vi "Autonomous Independent.vi"() -> ()   [LabVIEW 2017]
doc: "This VI is called when autonomous begins, and will automatically be terminated when autonomous ends. You can carry out timed or sensor driven robot movement independently without needing to return to the caller."
uses:
  <vilib>/Rock Robotics/WPI/ThirdParty/Sensors/navX/_TypeDefs/FRIC_navX_DeviceNumbersTypeDef.ctl
  <vilib>/Rock Robotics/WPI/Solenoid/WPI_SolenoidValue.ctl
  <vilib>/Rock Robotics/WPI/ThirdParty/Phoenix-LabVIEW/Motor Controller/Controls/CTRE_Phoenix_MotorControl_ControlMode.ctl
  <vilib>/Rock Robotics/WPI/Utilities/WPI_GetSetVariantRefNum.vi
  <vilib>/Rock Robotics/Network Tables/NT Read String.vi
  <vilib>/Rock Robotics/Network Tables/NT Write Numeric Array.vi
  <vilib>/Rock Robotics/WPI/Solenoid/WPI_SolenoidSetEnum.vi
panel:
  out "error out":errorcluster
  out "Array":dbl[](array[numeric])
  out "Direction":string[](array[string])
  in  "Target Angle":dbl format="%#_13g"
  in  "Target Distance":dbl=500.0 format="%#_13g"
  # "Be sure to right-click and choose Data Operations>>Make Current Value default if you want to save the array values with the VI"
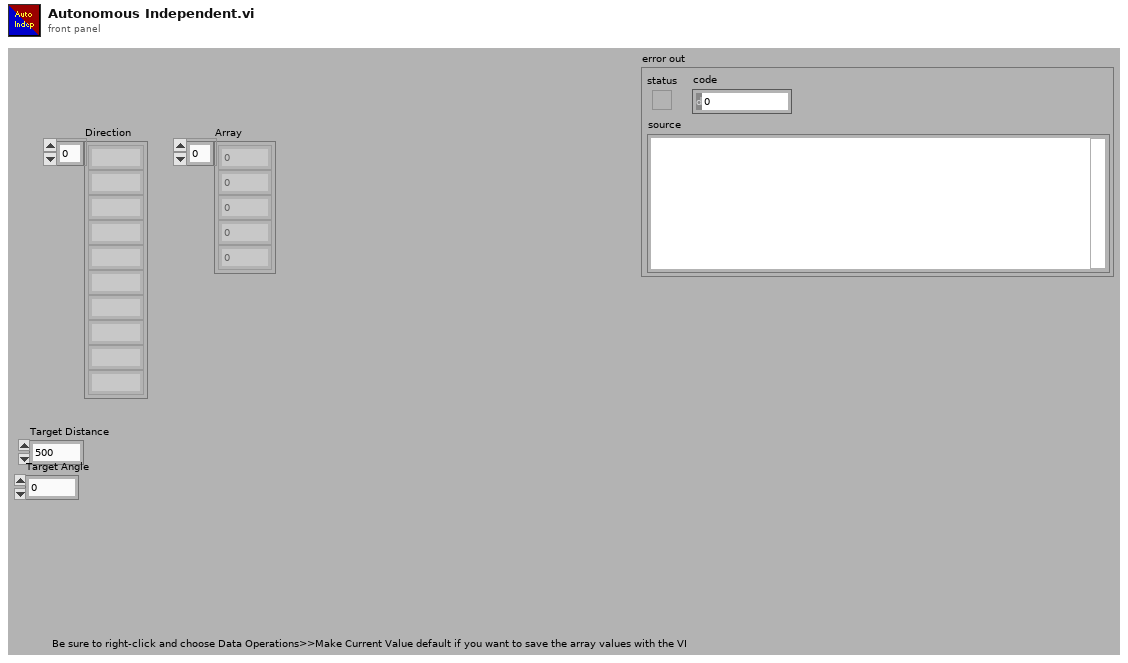
[diagram p1: front panel]
types:
  T1 = typedef "FRIC_navX_DeviceNumbersTypeDef.ctl" = enum16{"Dev0", "Dev1", "Dev2", "Dev3"}
  T2 = cluster{"Left Encoder":string, "Right Encoder":string, "Gyro Refnum":string, "Device Number":T1, "Right Refnum":string, "Left Refnum":string, "Right Intake":string, "Left Intake":string}
  T3 = typedef "WPI_JoystickDevRef.ctl" = cluster{"Device":T4}
  T4 = typedef "WPI_JoystickDeviceEnum.ctl" = enum16{"USB 0", "USB 1", "USB 2", "USB 3", "USB 4", "USB 5"}
  T5 = typedef "WPI_SolenoidValue.ctl" = enum16{"Off", "On", "Forward", "Reverse"}
  T6 = typedef "WPI_SolenoidDevRef.ctl" = cluster{"DevStatus":errorcluster, "Pneumatics Control Module":u8, "Forward Solenoid Channel":T7, "Reverse Solenoid Channel":T7}
  T7 = typedef "WPI_SolenoidChannel.ctl" = enum8{"Solenoid 0", "Solenoid 1", "Solenoid 2", "Solenoid 3", "Solenoid 4", "Solenoid 5", "Solenoid 6", "Solenoid 7", "Invalid"}
  T8 = cluster{"Left Encoder":string, "Right Encoder":string, "Gyro Refnum":string, "Device Number":T1, "Right Refnum":string, "Left Refnum":string}
  T9 = cluster{"Left Encoder":string, "Right Encoder":string, "Gyro Refnum":string, "Device Number":T1, "Right Refnum":string, "Left Refnum":string, "Left Intake":string, "Right Intake":string}
  T10 = typedef "CTRE_Phoenix_MotorControl_ControlMode.ctl" = u16
  T11 = typedef "WPI_MotorControlDeviceRef.ctl" = cluster{"DeviceStatus":errorcluster, "Type":T12, "PWM":cluster{"PWM Channel":T13, "DeadBand":T14}, "CAN":cluster{"Device Number":u8, "SetOutput VI Ref":variant, "GetOutput VI Ref":variant, "Enable VI Ref":variant, "Disable VI Ref":variant, "Data":variant}, "Invert":bool, "DIO PWM":cluster{"PWM \"Enable\" Channel":T13, "DIOChannel":T15, "PWM Rate":dbl}}
  T12 = typedef "WPI_MotorControlType.ctl" = enum16{"PWM", "CAN", "DIO PWM"}
  T13 = typedef "FPGA_DIOPWMChannel.ctl" = enum8{"PWM 0", "PWM 1", "PWM 2", "PWM 3", "PWM 4", "PWM 5", "PWM 6", "PWM 7", "PWM 8", "PWM 9", "PWM MXP 0", "PWM MXP 1", "PWM MXP 2", "PWM MXP 3", "PWM MXP 4", "PWM MXP 5", "PWM MXP 6", "PWM MXP 7", "PWM MXP 8", "PWM MXP 9", "Invalid"}
  T14 = typedef "WPI_PWMDeadband.ctl" = cluster{"Name":string, "maxPositivePwm":i32, "minPositivePwm":i32, "centerPwm":i32, "maxNegativePwm":i32, "minNegativePwm":i32, "angularRange":u16}
  T15 = typedef "FPGA_DIOChannel.ctl" = enum8{"DIO 0", "DIO 1", "DIO 2", "DIO 3", "DIO 4", "DIO 5", "DIO 6", "DIO 7", "DIO 8", "DIO 9", "DIO MXP 0", "DIO MXP 1", "DIO MXP 2", "DIO MXP 3", "DIO MXP 4", "DIO MXP 5", "DIO MXP 6", "DIO MXP 7", "DIO MXP 8", "DIO MXP 9", "DIO MXP 10", "DIO MXP 11", "DIO MXP 12", "DIO MXP 13", "DIO MXP 14", "DIO MXP 15", "SPI Port CS1", "SPI Port CS2", "SPI Port CS3", "SPI Port MISO", "SPI Port MOSI", "Invalid"}
  T16 = cluster{"Width":u16, "Style":enum32{"Solid", "Dash", "Dot", "DashDot", "DashDotDot"}}
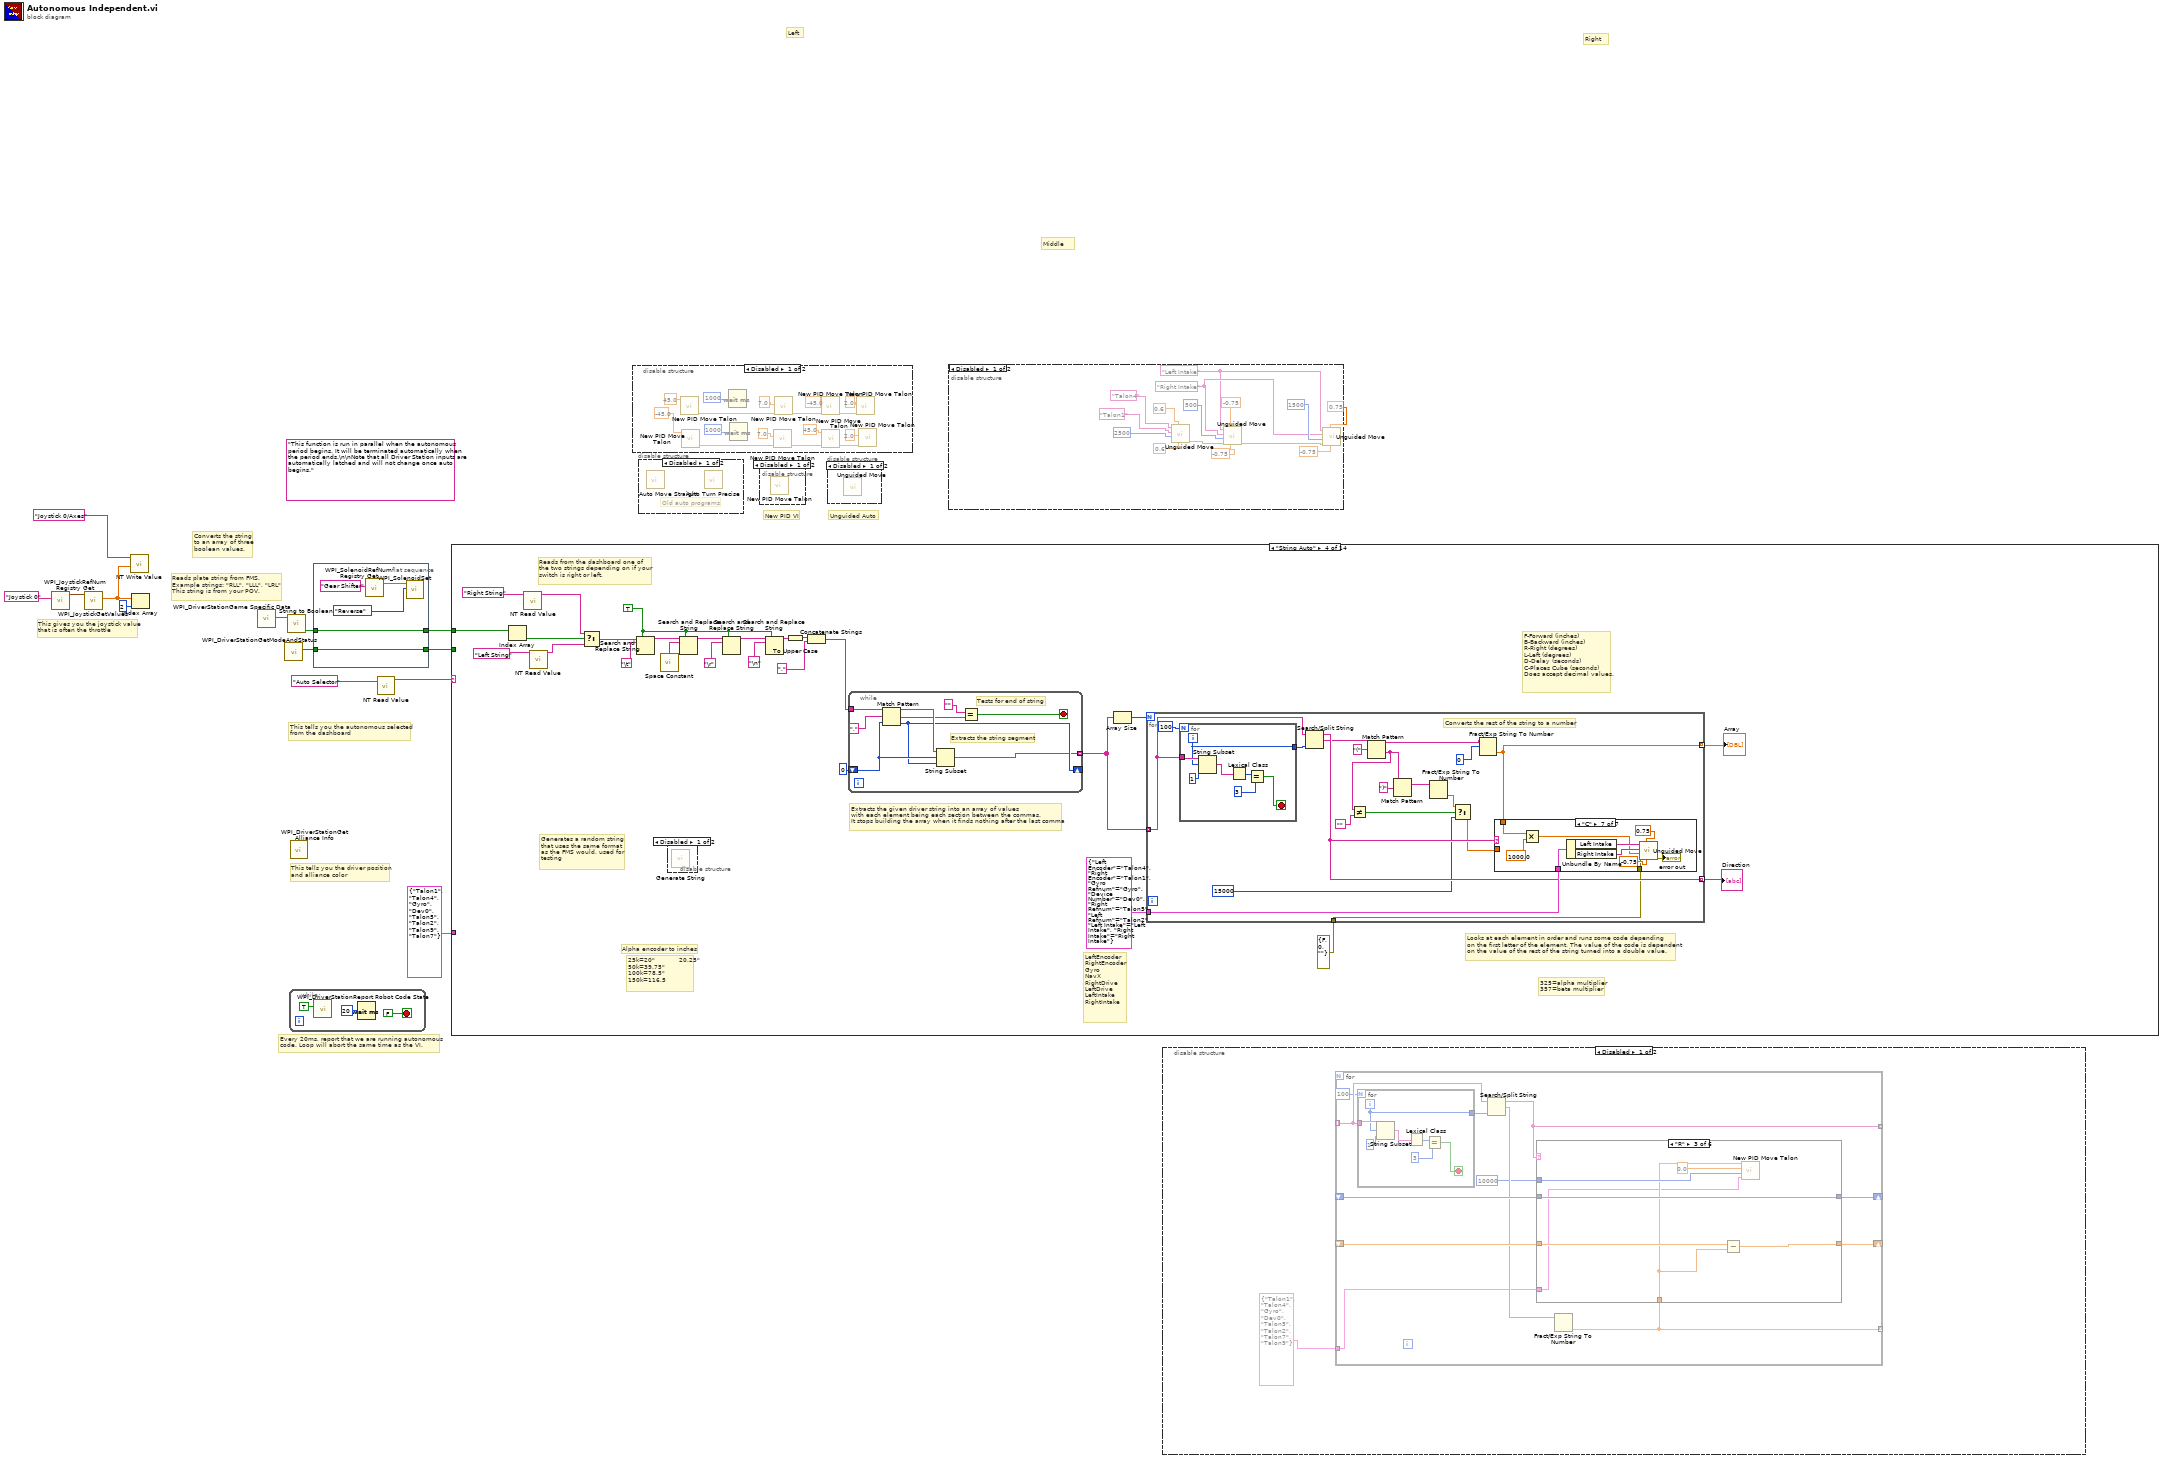
[diagram p0: block diagram]
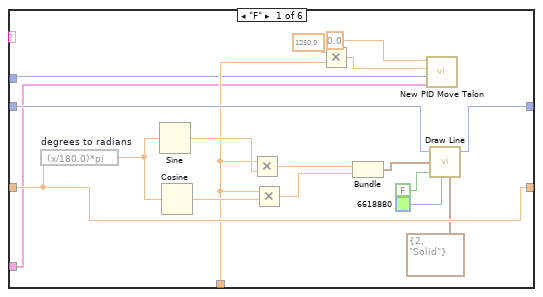
[diagram p2: hidden frame]
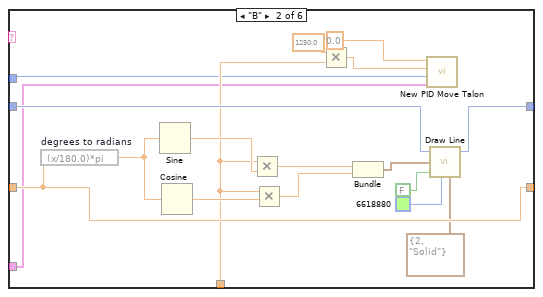
[diagram p3: hidden frame]
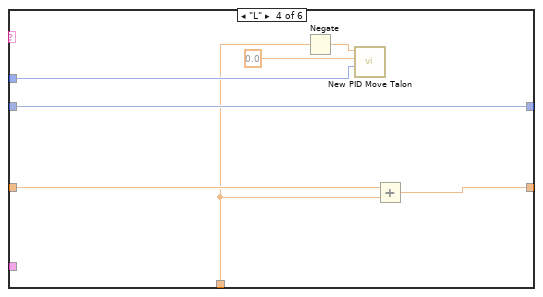
[diagram p4: hidden frame]
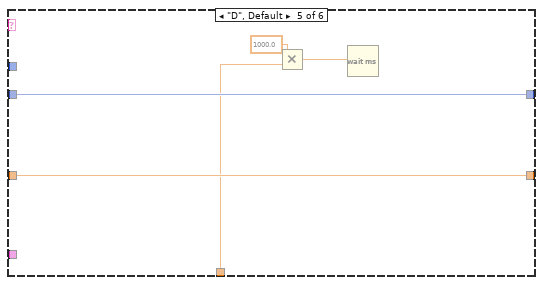
[diagram p5: hidden frame]
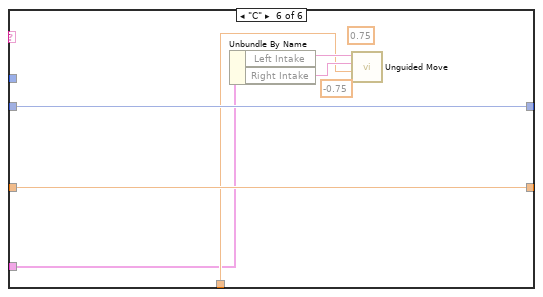
[diagram p6: hidden frame]
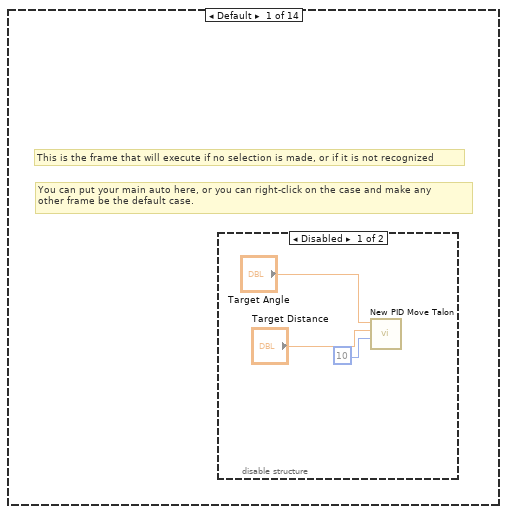
[diagram p13: hidden frame]
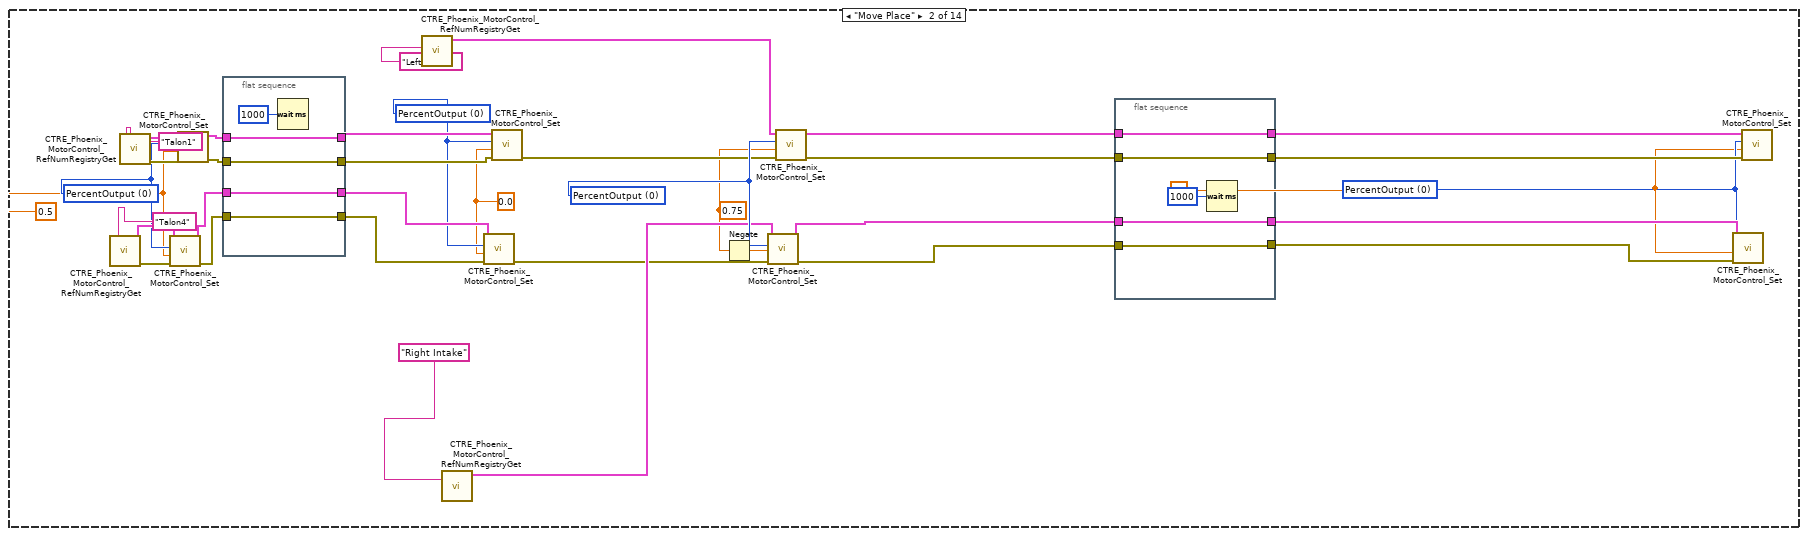
[diagram p15: hidden frame]
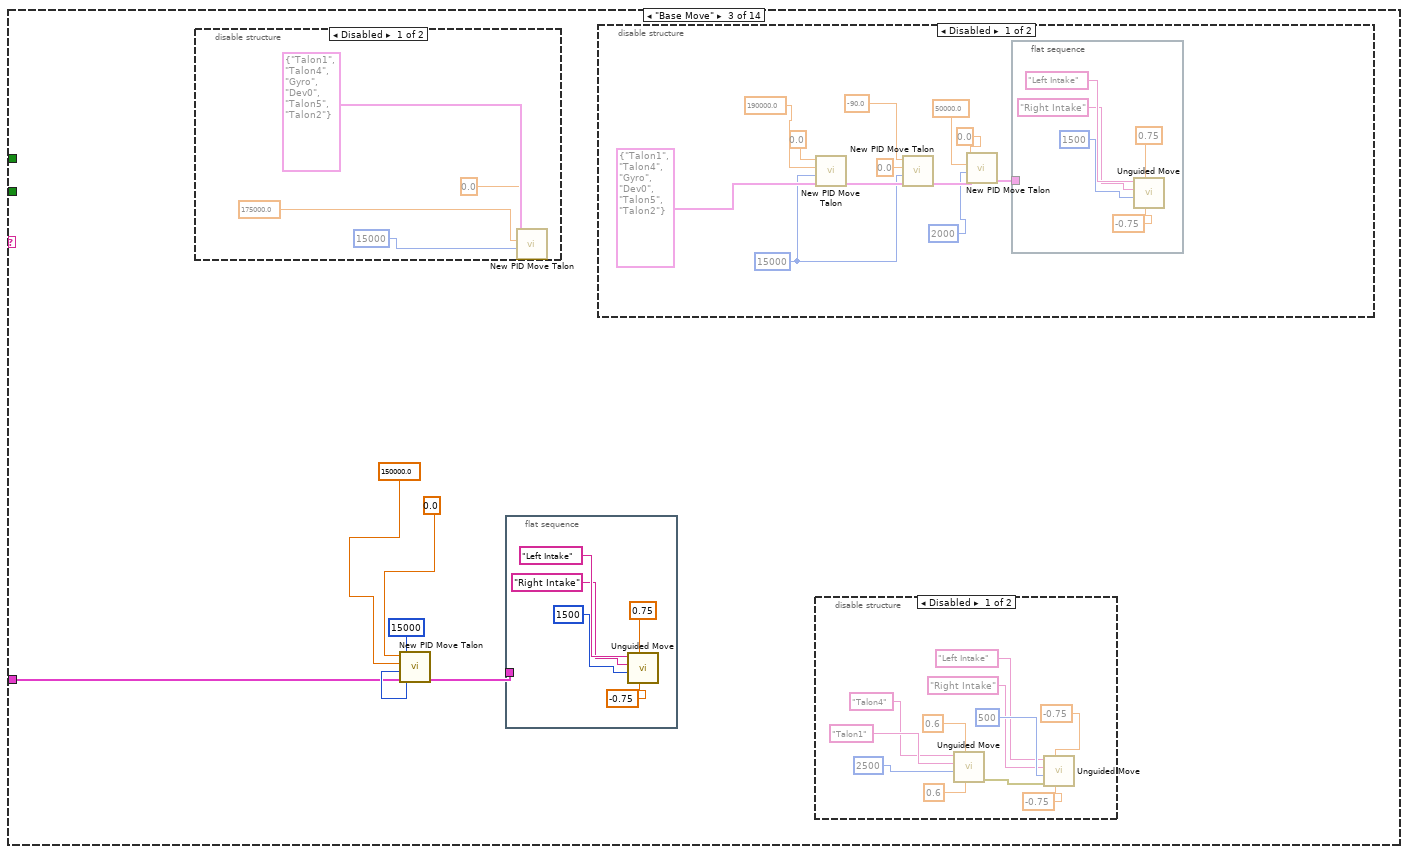
[diagram p16: hidden frame]
diagram:
  (unwired) "This function is run in parallel when the autonomous period begins. It will be terminated automatically when the period ends.\n\nNote that all Driver Station inputs are automatically latched and will not change once auto begins."
  # "Unguided Auto"
  # "New PID VI"
  # "Converts the string\nto an array of three\nboolean values."
  # "Reads plate string from FMS. \nExample strings: \"RLL\", \"LLL\", \"LRL\"\nThis string is from your POV."
  # "Middle"
  # "Left"
  # "Right"
  # "This tells you the autonomous selected\nfrom the dashboard"
  # "Every 20ms, report that we are running autonomous\ncode. Loop will abort the same time as the VI."
  # "This gives you the joystick value\nthat is often the throttle"
  # "This tells you the driver position\nand alliance color"
  n1 = call <vilib>:"WPI_JoystickRefNum Registry Get.vi"("refnum name"="Joystick 0") -> ("JoystickDevRef"=w12:T3)  [unwired: 1 in, 9 out]
  n2 = call <vilib>:"WPI_JoystickGetValues.vi"("JoystickDevRef"=w12) -> ("Axes"=w8:dbl[])  [unwired: 6 in, 4 out]
  n3 = call-poly <vilib>:"NT Write Value.vi"("Numeric Array"=w8, "Name"="Joystick 0/Axes") -> ()  [unwired: 9 in, 1 out]
  n4 = Index Array(array=w8, index=2) -> ()  [unwired: 1 out]
  n5 = call <vilib>:"WPI_DriverStationGame Specific Data.vi"() -> ("Game Specific Data"=w6:string)  [unwired: 11 in]
  n6 = call <vilib>:"WPI_DriverStationGetModeAndStatus.vi"() -> ("FMS Attached"=w1:bool)  [unwired: 10 in, 1 out]
  n7 = call "String to Boolean.vi"("String"=w6) -> ("Boolean Array"=w3:bool[])  [unwired: 10 in]
  n8 = while {
    stop <- FALSE stop-if-true
    n9 = call <vilib>:"WPI_DriverStationReport Robot Code State.vi"("Autonomous"=TRUE) -> ()  [unwired: 10 in, 1 out]
    n10 = Wait (ms)(milliseconds to wait=u32 20) -> ()  [unwired: 1 out]
  }
  n11 = call <vilib>:"WPI_DriverStationGet Alliance Info.vi"() -> ()  [unwired: 12 out]
  n12 = flat-sequence {
    tunnel: [w21] -> w4
    tunnel: w3 -> [w21]
    tunnel: [w17] -> w2
    tunnel: w1 -> [w17]
    frame #0 {
      n13 = call <vilib>:"WPI_SolenoidRefNum Registry Get.vi"("refnum name"="Gear Shifter") -> ("SolenoidDevRef"=w20:T6)  [unwired: 9 in, 1 out]
      n14 = call-poly <vilib>:"WPI_SolenoidSet.vi"("Value"=WPI_SolenoidValue."Reverse", "SolenoidDevRef"=w20) -> ()  [unwired: 8 in, 2 out]
    }
  }
  n15 = call-poly <vilib>:"NT Read Value.vi"("Name"="Auto Selector") -> ("String"=w9:string)  [unwired: 9 in, 1 out]
  n16 = case shown="\"String Auto\"" w9 {
    tunnel: w4 -> [_ _ _ w128 w212 _ _ w260 _ _ _ _ _ _]
    tunnel: T2 {"Left Encoder"="Talon1", "Right Encoder"="Talon4", "Gyro Refnum"="Gyro", "Device Number"=enum."Dev0", "Right Refnum"="Talon5", "Left Refnum"="Talon2", "Right Intake"="Talon9", "Left Intake"="Talon7"} ("Cluster 3") -> [_ _ w72 _ _ _ _ _ _ _ _ _ _ _]
    tunnel: w2 -> [_ _ _ _ _ _ _ _ _ _ _ _ _ _]
    frame Default {
      # "You can put your main auto here, or you can right-click on the case and make any\nother frame be the default case."
      # "This is the frame that will execute if no selection is made, or if it is not recognized"
      n17 = disable-structure shown="Disabled" {
        frame Disabled {
          n18 = call "New PID Move Talon.vi"("Timeout"=i8 10, "Target Distance"="Target Distance", "Target Angle"="Target Angle") -> ()  [unwired: 8 in, 1 out]
        }
        frame Enabled {
        }
      }
    }
    frame "Move Place" {
      w27 = 0.0 ("Output")
      w28 = T10 0 items=["PercentOutput"=0, "Position"=1, "Velocity"=2, "Current"=3, "Follower"=5, "MotionProfile"=6, "MotionMagic"=7, "MotionMagicArc"=8, "MotionProfileArc"=10, "Disabled"=15] ("Control Mode")
      w26 = 0.75 ("Output")
      w43 = T10 0 items=["PercentOutput"=0, "Position"=1, "Velocity"=2, "Current"=3, "Follower"=5, "MotionProfile"=6, "MotionMagic"=7, "MotionMagicArc"=8, "MotionProfileArc"=10, "Disabled"=15] ("Control Mode")
      w44 = 0.0 ("Output")
      w45 = T10 0 items=["PercentOutput"=0, "Position"=1, "Velocity"=2, "Current"=3, "Follower"=5, "MotionProfile"=6, "MotionMagic"=7, "MotionMagicArc"=8, "MotionProfileArc"=10, "Disabled"=15] ("Control Mode")
      w54 = 0.5 ("Output")
      w55 = T10 0 items=["PercentOutput"=0, "Position"=1, "Velocity"=2, "Current"=3, "Follower"=5, "MotionProfile"=6, "MotionMagic"=7, "MotionMagicArc"=8, "MotionProfileArc"=10, "Disabled"=15] ("Control Mode")
      n19 = call <vilib>:"CTRE_Phoenix_MotorControl_RefNumRegistryGet.vi"("refnum name"="Talon4") -> ("error out"=w56:errorcluster, "PhoenixMotorControlDevRef"=w57:T11)  [unwired: 9 in]
      n20 = call <vilib>:"CTRE_Phoenix_MotorControl_RefNumRegistryGet.vi"("refnum name"="Talon1") -> ("error out"=w59:errorcluster, "PhoenixMotorControlDevRef"=w58:T11)  [unwired: 9 in]
      n21 = call <vilib>:"CTRE_Phoenix_MotorControl_Set.vi"("error in (no error)"=w56, "Output"=w54, "Control Mode"=w55, "PhoenixMotorControlDevRef"=w57) -> ("error out"=w50:errorcluster, "PhoenixMotorControlDevRef"=w51:T11)  [unwired: 6 in]
      n22 = call <vilib>:"CTRE_Phoenix_MotorControl_Set.vi"("error in (no error)"=w59, "Output"=w54, "Control Mode"=w55, "PhoenixMotorControlDevRef"=w58) -> ("error out"=w52:errorcluster, "PhoenixMotorControlDevRef"=w53:T11)  [unwired: 6 in]
      n23 = flat-sequence {
        tunnel: w53 -> [w71]
        tunnel: [w71] -> w49
        tunnel: [w70] -> w47
        tunnel: w51 -> [w70]
        tunnel: [w69] -> w46
        tunnel: w50 -> [w69]
        tunnel: w52 -> [w68]
        tunnel: [w68] -> w48
        frame #0 {
          n24 = Wait (ms)(milliseconds to wait=u32 1000) -> ()  [unwired: 1 out]
        }
      }
      n25 = call <vilib>:"CTRE_Phoenix_MotorControl_RefNumRegistryGet.vi"("refnum name"="Left Intake") -> ("PhoenixMotorControlDevRef"=w42:T11)  [unwired: 9 in, 1 out]
      n26 = call <vilib>:"CTRE_Phoenix_MotorControl_RefNumRegistryGet.vi"("refnum name"="Right Intake") -> ("PhoenixMotorControlDevRef"=w41:T11)  [unwired: 9 in, 1 out]
      n27 = call <vilib>:"CTRE_Phoenix_MotorControl_Set.vi"("error in (no error)"=w46, "Output"=w44, "Control Mode"=w45, "PhoenixMotorControlDevRef"=w47) -> ("error out"=w40:errorcluster)  [unwired: 6 in, 1 out]
      n28 = call <vilib>:"CTRE_Phoenix_MotorControl_Set.vi"("error in (no error)"=w48, "Output"=w44, "Control Mode"=w45, "PhoenixMotorControlDevRef"=w49) -> ("error out"=w39:errorcluster)  [unwired: 6 in, 1 out]
      n29 = Negate(x=w26) -> (-x=w25:dbl)
      n30 = call <vilib>:"CTRE_Phoenix_MotorControl_Set.vi"("error in (no error)"=w40, "Output"=w25, "Control Mode"=w43, "PhoenixMotorControlDevRef"=w41) -> ("error out"=w36:errorcluster, "PhoenixMotorControlDevRef"=w33:T11)  [unwired: 6 in]
      n31 = call <vilib>:"CTRE_Phoenix_MotorControl_Set.vi"("error in (no error)"=w39, "Output"=w26, "Control Mode"=w43, "PhoenixMotorControlDevRef"=w42) -> ("error out"=w35:errorcluster, "PhoenixMotorControlDevRef"=w34:T11)  [unwired: 6 in]
      n32 = flat-sequence {
        tunnel: [w66] -> w29
        tunnel: w36 -> [w66]
        tunnel: [w65] -> w31
        tunnel: w35 -> [w65]
        tunnel: [w64] -> w32
        tunnel: w34 -> [w64]
        tunnel: [w63] -> w30
        tunnel: w33 -> [w63]
        frame #0 {
          n33 = Wait (ms)(milliseconds to wait=u32 1000) -> ()  [unwired: 1 out]
        }
      }
      n34 = call <vilib>:"CTRE_Phoenix_MotorControl_Set.vi"("error in (no error)"=w29, "Output"=w27, "Control Mode"=w28, "PhoenixMotorControlDevRef"=w30) -> ()  [unwired: 6 in, 2 out]
      n35 = call <vilib>:"CTRE_Phoenix_MotorControl_Set.vi"("error in (no error)"=w31, "Output"=w27, "Control Mode"=w28, "PhoenixMotorControlDevRef"=w32) -> ()  [unwired: 6 in, 2 out]
    }
    frame "Base Move" {
      n36 = disable-structure shown="Disabled" {
        frame Disabled {
          n37 = call "New PID Move Talon.vi"("Cluster 3"=T8 {"Left Encoder"="Talon1", "Right Encoder"="Talon4", "Gyro Refnum"="Gyro", "Device Number"=enum."Dev0", "Right Refnum"="Talon5", "Left Refnum"="Talon2"}, "Timeout"=i16 15000, "Target Distance"=175000.0 ("Target Distance 2"), "Target Angle"=0.0) -> ()  [unwired: 7 in, 1 out]
        }
        frame Enabled {
        }
      }
      n38 = call "New PID Move Talon.vi"("Cluster 3"=w72, "Timeout"=i16 15000, "Target Distance"=150000.0, "Target Angle"=0.0) -> ("Cluster 2"=w73:T2)  [unwired: 7 in]
      n39 = flat-sequence {
        tunnel: w73 -> [_]
        frame #0 {
          n40 = call "Unguided Move.vi"("Power 2"=-0.75 ("Power"), "Power"=0.75, "milliseconds to wait"=u32 1500, "refnum name 2"="Right Intake" ("refnum name"), "refnum name"="Left Intake") -> ()  [unwired: 6 in, 1 out]
        }
      }
      n41 = disable-structure shown="Disabled" {
        frame Disabled {
          w89 = i16 15000 ("Timeout")
          n42 = call "New PID Move Talon.vi"("Cluster 3"=T8 {"Left Encoder"="Talon1", "Right Encoder"="Talon4", "Gyro Refnum"="Gyro", "Device Number"=enum."Dev0", "Right Refnum"="Talon5", "Left Refnum"="Talon2"}, "Timeout"=w89, "Target Distance"=190000.0, "Target Angle"=0.0) -> ("Cluster 2"=w93:T2)  [unwired: 7 in]
          n43 = call "New PID Move Talon.vi"("Cluster 3"=w93, "Timeout"=w89, "Target Distance"=0.0, "Target Angle"=-90.0) -> ("Cluster 2"=w92:T2)  [unwired: 7 in]
          n44 = call "New PID Move Talon.vi"("Cluster 3"=w92, "Timeout"=i16 2000, "Target Distance"=50000.0, "Target Angle"=0.0) -> ("Cluster 2"=w91:T2)  [unwired: 7 in]
          n45 = flat-sequence {
            tunnel: w91 -> [_]
            frame #0 {
              n46 = call "Unguided Move.vi"("Power 2"=-0.75 ("Power"), "Power"=0.75, "milliseconds to wait"=u32 1500, "refnum name 2"="Right Intake" ("refnum name"), "refnum name"="Left Intake") -> ()  [unwired: 6 in, 1 out]
            }
          }
        }
        frame Enabled {
        }
      }
      n47 = disable-structure shown="Disabled" {
        frame Disabled {
          n48 = call "Unguided Move.vi"("Power 2"=0.6, "Power"=0.6, "milliseconds to wait"=u32 2500, "refnum name 2"="Talon1", "refnum name"="Talon4") -> ("error out"=w109:errorcluster)  [unwired: 6 in]
          n49 = call "Unguided Move.vi"("Power 2"=-0.75 ("Power"), "Power"=-0.75, "error in (no error)"=w109, "milliseconds to wait"=u32 500, "refnum name 2"="Right Intake" ("refnum name"), "refnum name"="Left Intake") -> ()  [unwired: 5 in, 1 out]
        }
        frame Enabled {
        }
      }
    }
    frame "String Auto" {
      w120 = TRUE ("replace all? (F)")
      # "325=alpha multiplier\n357=beta multiplier"
      # "F-Forward (inches)\nB-Backward (inches)\nR-Right (degrees)\nL-Left (degrees)\nD-Delay (seconds)\nC-Places Cube (seconds)\nDoes accept decimal values."
      # "Alpha encoder to inches"
      # "LeftEncoder\nRightEncoder\nGyro\nNavX\nRightDrive\nLeftDrive\nLeftIntake\nRightIntake"
      # "25k=20\"            20.25\"\n50k=39.75\"\n100k=78.5\"\n150k=116.5"
      # "Looks at each element in order and runs some code depending\non the first letter of the element. The value of the code is dependent\non the value of the rest of the string turned into a double value."
      # "Extracts the given driver string into an array of values \nwith each element being each section between the commas.\nIt stops building the array when it finds nothing after the last comma"
      # "Reads from the dashboard one of\nthe two strings depending on if your\nswitch is right or left."
      # "Generates a random string\nthat uses the same format \nas the FMS would, used for\ntesting"
      n50 = Index Array(array=w128) -> (element=w139:bool)  [unwired: 1 in]
      n51 = call-poly <vilib>:"NT Read Value.vi"("Name"="Right String") -> ("String"=w138:string)  [unwired: 9 in, 1 out]
      n52 = call-poly <vilib>:"NT Read Value.vi"("Name"="Left String") -> ("String"=w135:string)  [unwired: 9 in, 1 out]
      n53 = Select(t=w138, s=w139, f=w135) -> (s? t:f=w118:string)
      n54 = Search and Replace String(replace all?=w120, input string=w118, search string="\t") -> (result string=w124:string)  [unwired: 5 in, 3 out]
      n55 = call <vilib>:"Space Constant.vi"() -> ("String"=w122:string)
      n56 = disable-structure shown="Disabled" {
        frame Disabled {
          n57 = call "Generate String.vi"() -> ()  [unwired: 11 in, 1 out]
        }
        frame Enabled {
        }
      }
      n58 = Search and Replace String(replace all?=w120, input string=w124, search string=w122) -> (result string=w125:string)  [unwired: 5 in, 3 out]
      n59 = Search and Replace String(replace all?=w120, input string=w125, search string="\r") -> (result string=w126:string)  [unwired: 5 in, 3 out]
      n60 = Search and Replace String(replace all?=w120, input string=w126, search string="\n") -> (result string=w119:string)  [unwired: 5 in, 3 out]
      n61 = To Upper Case(1:w119) -> (0:w116:string)
      n62 = Concatenate Strings(w116, "," ("regular expression")) -> (w115:string)
      n63 = while {
        tunnel: w115 -> [w209]
        shift-right: [w205] -> _
        shift-left: 0 ("offset past match") -> [w206]
        tunnel: [w204] -> w132 mode=indexing
        stop <- w201 stop-if-true
        # "Tests for end of string"
        # "Extracts the string segment"
        n64 = Match Pattern(string=w209, regular expression=",", offset (0)=w206) -> (before substring=w207:string, after substring=w203:string, offset past match=w205:i32)  [unwired: 1 out]
        n65 = String Subset(string=w207, offset (0)=w206, length (rest)=w205) -> (substring=w204:string)
        n66 = Equal?(x="", y=w203) -> (x = y?=w201:bool)
      }
      n67 = Array Size(array=w132) -> (size(s)=w133:i32)
      n68 = for {
        N: w133 -> [_]
        tunnel: w132 -> [w154] mode=indexing
        tunnel: [w157] -> w130 mode=indexing
        tunnel: [w153] -> w131 mode=indexing
        tunnel: T9 {"Left Encoder"="Talon4", "Right Encoder"="Talon1", "Gyro Refnum"="Gyro", "Device Number"=enum."Dev0", "Right Refnum"="Talon5", "Left Refnum"="Talon2", "Left Intake"="Left Intake", "Right Intake"="Right Intake"} ("Cluster 3") -> [w156]
        tunnel: errorcluster {"status"=FALSE, "code"=0, "source"=""} ("error in (no error)") -> [w151]
        # "Converts the rest of the string to a number"
        n69 = for {
          N: 100 -> [_]
          tunnel: w154 -> [w163]
          tunnel: [w160] -> w155
          i -> [w160]
          stop <- w159 stop-if-true
          n70 = String Subset(string=w163, offset (0)=w160, length (rest)=1 ("length (rest)")) -> (substring=w161:string)
          n71 = Lexical Class(1:w161) -> (0:w165:i16)
          n72 = Equal?(x=w165, y=i16 3) -> (x = y?=w159:bool)
        }
        n73 = Search/Split String(string=w154, offset (0)=w155) -> (substring before match=w153:string, match + rest of string=w150:string)  [unwired: 1 in, 1 out]
        n74 = Match Pattern(string=w150, regular expression="(") -> (before substring=w148:string, after substring=w144:string)  [unwired: 1 in, 2 out]
        n75 = Not Equal?(x=w144, y="") -> (x != y?=w143:bool)
        n76 = Match Pattern(string=w144, regular expression=")") -> (before substring=w147:string)  [unwired: 1 in, 3 out]
        n77 = Fract/Exp String To Number(string=w147) -> (number=w142:dbl)  [unwired: 3 in, 1 out]
        n78 = Select(t=w142, s=w143, f=i16 15000 ("Timeout")) -> (s? t:f=w140:dbl)
        n79 = Fract/Exp String To Number(string=w148, offset=0) -> (number=w157:dbl)  [unwired: 2 in, 1 out]
        n80 = case shown="\"C\"" w153 {
          tunnel: w157 -> [_ w167 w175 w182 w185 w189 w199]
          tunnel: w156 -> [_ w171 w178 w180 w184 _ w200]
          tunnel: w140 -> [_ w170 w177 w179 w183 _ _]
          tunnel: w151 -> [_ _ _ _ _ _ w191]
          frame "\u0000", Default {
          }
          frame "F" {
            n81 = Multiply(x=1250.0, y=w167) -> (x*y=w166:dbl)
            n82 = call "New PID Move Talon.vi"("Cluster 3"=w171, "Timeout"=w170, "Target Distance"=w166, "Target Angle"=0.0) -> ()  [unwired: 7 in, 1 out]
          }
          frame "B" {
            n83 = Negate(x=w175) -> (-x=w174:dbl)
            n84 = Multiply(x=1250.0, y=w174) -> (x*y=w173:dbl)
            n85 = call "New PID Move Talon.vi"("Cluster 3"=w178, "Timeout"=w177, "Target Distance"=w173, "Target Angle"=0.0) -> ()  [unwired: 7 in, 1 out]
          }
          frame "R" {
            n86 = call "New PID Move Talon.vi"("Cluster 3"=w180, "Timeout"=w179, "Target Distance"=0.0, "Target Angle"=w182) -> ()  [unwired: 7 in, 1 out]
          }
          frame "L" {
            n87 = Negate(x=w185) -> (-x=w186:dbl)
            n88 = call "New PID Move Talon.vi"("Cluster 3"=w184, "Timeout"=w183, "Target Distance"=0.0, "Target Angle"=w186) -> ()  [unwired: 7 in, 1 out]
          }
          frame "D" {
            n89 = Multiply(x=1000.0, y=w189) -> (x*y=w188:dbl)
            n90 = Wait (ms)(milliseconds to wait=w188) -> ()  [unwired: 1 out]
          }
          frame "C" {
            n91 = Multiply(x=w199, y=1000.0) -> (x*y=w195:dbl)
            n92 = Unbundle By Name(w200) -> ("Left Intake"=w196:string, "Right Intake"=w197:string)
            n93 = call "Unguided Move.vi"("Power 2"=-0.75, "Power"=0.75, "error in (no error)"=w191, "milliseconds to wait"=w195, "refnum name 2"=w197, "refnum name"=w196) -> ("error out"=→"error out":errorcluster)  [unwired: 5 in]
          }
        }
      }
      "Direction" <- w131
      "Array" <- w130
    }
    frame "Front Left Auto" {
      w215 = "Right Intake" ("refnum name")
      w213 = "Left Intake" ("refnum name")
      n94 = Index Array(array=w212) -> (element=w211:bool)  [unwired: 1 in]
      n95 = Not(x=w211) -> (.not. x?=w210:bool)
      n96 = call "Unguided Move.vi"("Power 2"=0.6, "Power"=0.6, "milliseconds to wait"=u32 2500, "refnum name 2"="Talon1", "refnum name"="Talon4") -> ("error out"=w217:errorcluster)  [unwired: 6 in]
      n97 = call "Unguided Move.vi"("Power 2"=-0.75 ("Power"), "Power"=-0.75, "error in (no error)"=w217, "milliseconds to wait"=u32 500, "refnum name 2"=w215, "refnum name"=w213) -> ("error out"=w214:errorcluster)  [unwired: 5 in]
      n98 = case shown="True" w210 {
        tunnel: w215 -> [_ w230]
        tunnel: w214 -> [_ w227]
        tunnel: w213 -> [_ w226]
        frame False {
        }
        frame True {
          n99 = call "Unguided Move.vi"("Power 2"=-0.75, "Power"=0.75, "error in (no error)"=w227, "milliseconds to wait"=u32 1500, "refnum name 2"=w230, "refnum name"=w226) -> ()  [unwired: 5 in, 1 out]
        }
      }
      n100 = disable-structure shown="Disabled" {
        frame Disabled {
          n101 = call "New PID Move Talon.vi"("Target Distance"=4.0 ("Target Angle")) -> ("Cluster 2"=w237:T2)  [unwired: 10 in]
          n102 = call "New PID Move Talon.vi"("Cluster 3"=w237, "Target Angle"=90.0 ("Target Distance")) -> ("Cluster 2"=w238:T2)  [unwired: 9 in]
          n103 = call "New PID Move Talon.vi"("Cluster 3"=w238, "Target Distance"=5.0 ("Target Angle")) -> ("Cluster 2"=w236:T2)  [unwired: 9 in]
          n104 = call "New PID Move Talon.vi"("Cluster 3"=w236, "Target Angle"=-90.0 ("Target Distance")) -> ("Cluster 2"=w239:T2)  [unwired: 9 in]
          n105 = call "New PID Move Talon.vi"("Cluster 3"=w239, "Target Distance"=5.0) -> ()  [unwired: 9 in, 1 out]
        }
        frame Enabled {
        }
      }
    }
    frame "Side Left Auto" {
      w240 = i16 15000 ("Timeout")
      n106 = call "New PID Move Talon.vi"("Timeout"=w240, "Target Distance"=150000.0) -> ("Cluster 2"=w245:T2)  [unwired: 9 in]
      n107 = call "New PID Move Talon.vi"("Cluster 3"=w245, "Timeout"=w240, "Target Angle"=90.0) -> ("Cluster 2"=w244:T2)  [unwired: 8 in]
      n108 = call "New PID Move Talon.vi"("Cluster 3"=w244, "Timeout"=w240, "Target Distance"=10000.0) -> ()  [unwired: 8 in, 1 out]
    }
    frame "Other Side Left Auto" {
      n109 = call "New PID Move Talon.vi"("Target Distance"=18.5 ("Target Angle")) -> ("Cluster 2"=w254:T2)  [unwired: 10 in]
      n110 = call "New PID Move Talon.vi"("Cluster 3"=w254, "Target Angle"=90.0 ("Target Distance")) -> ("Cluster 2"=w255:T2)  [unwired: 9 in]
      n111 = call "New PID Move Talon.vi"("Cluster 3"=w255, "Target Distance"=18.0 ("Target Angle")) -> ("Cluster 2"=w253:T2)  [unwired: 9 in]
      n112 = call "New PID Move Talon.vi"("Cluster 3"=w253, "Target Angle"=90.0 ("Target Distance")) -> ("Cluster 2"=w256:T2)  [unwired: 9 in]
      n113 = call "New PID Move Talon.vi"("Cluster 3"=w256, "Target Distance"=5.0) -> ("Cluster 2"=w257:T2)  [unwired: 9 in]
      n114 = call "New PID Move Talon.vi"("Cluster 3"=w257, "Target Angle"=90.0) -> ("Cluster 2"=w258:T2)  [unwired: 9 in]
      n115 = call "New PID Move Talon.vi"("Cluster 3"=w258, "Target Distance"=1.0) -> ()  [unwired: 9 in, 1 out]
    }
    frame "Front Right Auto" {
      w263 = "Right Intake" ("refnum name")
      w261 = "Left Intake" ("refnum name")
      n116 = Index Array(array=w260) -> (element=w259:bool)  [unwired: 1 in]
      n117 = call "Unguided Move.vi"("Power 2"=0.6, "Power"=0.6, "milliseconds to wait"=u32 2500, "refnum name 2"="Talon2", "refnum name"="Talon5") -> ("error out"=w265:errorcluster)  [unwired: 6 in]
      n118 = call "Unguided Move.vi"("Power 2"=-0.75 ("Power"), "Power"=-0.75, "error in (no error)"=w265, "milliseconds to wait"=u32 500, "refnum name 2"=w263, "refnum name"=w261) -> ("error out"=w262:errorcluster)  [unwired: 5 in]
      n119 = case shown="True" w259 {
        tunnel: w263 -> [_ w278]
        tunnel: w262 -> [_ w275]
        tunnel: w261 -> [_ w274]
        frame False {
        }
        frame True {
          n120 = call "Unguided Move.vi"("Power 2"=-0.75, "Power"=0.75, "error in (no error)"=w275, "milliseconds to wait"=u32 1500, "refnum name 2"=w278, "refnum name"=w274) -> ()  [unwired: 5 in, 1 out]
        }
      }
      n121 = disable-structure shown="Disabled" {
        frame Disabled {
          n122 = call "New PID Move Talon.vi"("Target Distance"=4.0 ("Target Angle")) -> ("Cluster 2"=w285:T2)  [unwired: 10 in]
          n123 = call "New PID Move Talon.vi"("Cluster 3"=w285, "Target Angle"=-90.0 ("Target Distance")) -> ("Cluster 2"=w286:T2)  [unwired: 9 in]
          n124 = call "New PID Move Talon.vi"("Cluster 3"=w286, "Target Distance"=5.0 ("Target Angle")) -> ("Cluster 2"=w284:T2)  [unwired: 9 in]
          n125 = call "New PID Move Talon.vi"("Cluster 3"=w284, "Target Angle"=90.0 ("Target Distance")) -> ("Cluster 2"=w287:T2)  [unwired: 9 in]
          n126 = call "New PID Move Talon.vi"("Cluster 3"=w287, "Target Distance"=5.0) -> ()  [unwired: 9 in, 1 out]
        }
        frame Enabled {
        }
      }
    }
    frame "Side Right Auto" {
      n127 = call "New PID Move Talon.vi"("Target Distance"=12.0) -> ("Cluster 2"=w292:T2)  [unwired: 10 in]
      n128 = call "New PID Move Talon.vi"("Cluster 3"=w292, "Target Angle"=-90.0) -> ("Cluster 2"=w291:T2)  [unwired: 9 in]
      n129 = call "New PID Move Talon.vi"("Cluster 3"=w291, "Target Distance"=1.5) -> ()  [unwired: 9 in, 1 out]
    }
    frame "Other Side Right Auto" {
      n130 = call "New PID Move Talon.vi"("Target Distance"=18.5 ("Target Angle")) -> ("Cluster 2"=w301:T2)  [unwired: 10 in]
      n131 = call "New PID Move Talon.vi"("Cluster 3"=w301, "Target Angle"=-90.0 ("Target Distance")) -> ("Cluster 2"=w302:T2)  [unwired: 9 in]
      n132 = call "New PID Move Talon.vi"("Cluster 3"=w302, "Target Distance"=18.0 ("Target Angle")) -> ("Cluster 2"=w300:T2)  [unwired: 9 in]
      n133 = call "New PID Move Talon.vi"("Cluster 3"=w300, "Target Angle"=-90.0 ("Target Distance")) -> ("Cluster 2"=w303:T2)  [unwired: 9 in]
      n134 = call "New PID Move Talon.vi"("Cluster 3"=w303, "Target Distance"=5.0) -> ("Cluster 2"=w304:T2)  [unwired: 9 in]
      n135 = call "New PID Move Talon.vi"("Cluster 3"=w304, "Target Angle"=-90.0) -> ("Cluster 2"=w305:T2)  [unwired: 9 in]
      n136 = call "New PID Move Talon.vi"("Cluster 3"=w305, "Target Distance"=1.0) -> ()  [unwired: 9 in, 1 out]
    }
    frame "Middle Left Side Auto" {
      n137 = call "New PID Move Talon.vi"("Target Distance"=5.0) -> ("Cluster 2"=w312:T2)  [unwired: 10 in]
      n138 = call "New PID Move Talon.vi"("Cluster 3"=w312, "Target Angle"=-90.0) -> ("Cluster 2"=w313:T2)  [unwired: 9 in]
      n139 = call "New PID Move Talon.vi"("Cluster 3"=w313, "Target Distance"=13.0) -> ("Cluster 2"=w314:T2)  [unwired: 9 in]
      n140 = call "New PID Move Talon.vi"("Cluster 3"=w314, "Target Distance"=7.0 ("Target Angle")) -> ("Cluster 2"=w315:T2)  [unwired: 9 in]
      n141 = call "New PID Move Talon.vi"("Cluster 3"=w315, "Target Angle"=90.0 ("Target Distance")) -> ("Cluster 2"=w316:T2)  [unwired: 9 in]
      n142 = call "New PID Move Talon.vi"("Cluster 3"=w316, "Target Distance"=1.0) -> ()  [unwired: 9 in, 1 out]
    }
    frame "Middle Right Front Auto" {
      n143 = call "New PID Move Talon.vi"("Target Distance"=9.0) -> ()  [unwired: 10 in, 1 out]
    }
    frame "Middle Right Side Auto" {
      n144 = call "New PID Move Talon.vi"("Target Distance"=6.0) -> ("Cluster 2"=w325:T2)  [unwired: 10 in]
      n145 = call "New PID Move Talon.vi"("Cluster 3"=w325, "Target Angle"=90.0) -> ("Cluster 2"=w326:T2)  [unwired: 9 in]
      n146 = call "New PID Move Talon.vi"("Cluster 3"=w326, "Target Distance"=4.0) -> ("Cluster 2"=w327:T2)  [unwired: 9 in]
      n147 = call "New PID Move Talon.vi"("Cluster 3"=w327, "Target Angle"=-90.0) -> ("Cluster 2"=w328:T2)  [unwired: 9 in]
      n148 = call "New PID Move Talon.vi"("Cluster 3"=w328, "Target Distance"=7.0) -> ("Cluster 2"=w329:T2)  [unwired: 9 in]
      n149 = call "New PID Move Talon.vi"("Cluster 3"=w329, "Target Angle"=-90.0) -> ("Cluster 2"=w330:T2)  [unwired: 9 in]
      n150 = call "New PID Move Talon.vi"("Cluster 3"=w330, "Target Distance"=1.0) -> ()  [unwired: 9 in, 1 out]
    }
    frame "Middle Left Front Auto" {
      n151 = call "New PID Move Talon.vi"("Target Distance"=4.0) -> ("Cluster 2"=w336:T2)  [unwired: 10 in]
      n152 = call "New PID Move Talon.vi"("Cluster 3"=w336, "Target Angle"=-90.0) -> ("Cluster 2"=w337:T2)  [unwired: 9 in]
      n153 = call "New PID Move Talon.vi"("Cluster 3"=w337, "Target Distance"=9.0) -> ("Cluster 2"=w338:T2)  [unwired: 9 in]
      n154 = call "New PID Move Talon.vi"("Cluster 3"=w338, "Target Angle"=90.0) -> ("Cluster 2"=w339:T2)  [unwired: 9 in]
      n155 = call "New PID Move Talon.vi"("Cluster 3"=w339, "Target Distance"=5.0) -> ()  [unwired: 9 in, 1 out]
    }
  }
  n156 = disable-structure shown="Disabled" {
    frame Disabled {
      n157 = call "New PID Move Talon.vi"("Target Angle"=45.0) -> ("Cluster 2"=w350:T2)  [unwired: 10 in]
      n158 = call "New PID Move Talon.vi"("Target Angle"=-45.0) -> ("Cluster 2"=w343:T2)  [unwired: 10 in]
      n159 = Wait (ms)(milliseconds to wait=u32 1000) -> ()  [unwired: 1 out]
      n160 = Wait (ms)(milliseconds to wait=u32 1000) -> ()  [unwired: 1 out]
      n161 = call "New PID Move Talon.vi"("Cluster 3"=w343, "Target Distance"=7.0) -> ("Cluster 2"=w342:T2)  [unwired: 9 in]
      n162 = call "New PID Move Talon.vi"("Cluster 3"=w350, "Target Distance"=7.0) -> ("Cluster 2"=w349:T2)  [unwired: 9 in]
      n163 = call "New PID Move Talon.vi"("Cluster 3"=w349, "Target Angle"=-45.0) -> ("Cluster 2"=w348:T2)  [unwired: 9 in]
      n164 = call "New PID Move Talon.vi"("Cluster 3"=w342, "Target Angle"=45.0) -> ("Cluster 2"=w341:T2)  [unwired: 9 in]
      n165 = call "New PID Move Talon.vi"("Cluster 3"=w348, "Target Distance"=2.0) -> ()  [unwired: 9 in, 1 out]
      n166 = call "New PID Move Talon.vi"("Cluster 3"=w341, "Target Distance"=2.0) -> ()  [unwired: 9 in, 1 out]
    }
    frame Enabled {
    }
  }
  n167 = disable-structure shown="Disabled" {
    frame Disabled {
      # "Old auto programs"
      n168 = call "Auto Move Straight.vi"() -> ()  [unwired: 10 in, 2 out]
      n169 = call "Auto Turn Precise.vi"() -> ()  [unwired: 10 in, 2 out]
    }
    frame Enabled {
    }
  }
  n170 = disable-structure shown="Disabled" {
    frame Disabled {
      n171 = call "New PID Move Talon.vi"() -> ()  [unwired: 11 in, 1 out]
    }
    frame Enabled {
    }
  }
  n172 = disable-structure shown="Disabled" {
    frame Disabled {
      n173 = call "Unguided Move.vi"() -> ()  [unwired: 11 in, 1 out]
    }
    frame Enabled {
    }
  }
  n174 = disable-structure shown="Disabled" {
    frame Disabled {
      w366 = "Right Intake" ("refnum name")
      w365 = "Left Intake" ("refnum name")
      n175 = call "Unguided Move.vi"("Power 2"=0.6, "Power"=0.6, "milliseconds to wait"=u32 2500, "refnum name 2"="Talon1", "refnum name"="Talon4") -> ("error out"=w363:errorcluster)  [unwired: 6 in]
      n176 = call "Unguided Move.vi"("Power 2"=-0.75 ("Power"), "Power"=-0.75, "error in (no error)"=w363, "milliseconds to wait"=u32 500, "refnum name 2"=w366, "refnum name"=w365) -> ("error out"=w370:errorcluster)  [unwired: 5 in]
      n177 = call "Unguided Move.vi"("Power 2"=-0.75, "Power"=0.75, "error in (no error)"=w370, "milliseconds to wait"=u32 1500, "refnum name 2"=w366, "refnum name"=w365) -> ()  [unwired: 5 in, 1 out]
    }
    frame Enabled {
    }
  }
  n178 = disable-structure shown="Disabled" {
    frame Disabled {
      n179 = for {
        tunnel: [w383] -> _ mode=indexing
        tunnel: [w376] -> _ mode=indexing
        tunnel: _ -> [w377] mode=indexing
        shift-right: [w381] -> _
        shift-left: _ -> [w382]
        shift-right: [w379] -> _
        shift-left: _ -> [w380]
        tunnel: T9 {"Left Encoder"="Talon1", "Right Encoder"="Talon4", "Gyro Refnum"="Gyro", "Device Number"=enum."Dev0", "Right Refnum"="Talon5", "Left Refnum"="Talon2", "Left Intake"="Talon7", "Right Intake"="Talon9"} ("Cluster 3") -> [w372]
        n180 = for {
          N: 100 -> [_]
          tunnel: w377 -> [w449]
          tunnel: [w446] -> w378
          i -> [w446]
          stop <- w445 stop-if-true
          n181 = String Subset(string=w449, offset (0)=w446, length (rest)=1 ("length (rest)")) -> (substring=w447:string)
          n182 = Lexical Class(1:w447) -> (0:w451:i16)
          n183 = Equal?(x=w451, y=i16 3) -> (x = y?=w445:bool)
        }
        n184 = Search/Split String(string=w377, offset (0)=w378) -> (substring before match=w376:string, match + rest of string=w375:string)  [unwired: 1 in, 1 out]
        n185 = Fract/Exp String To Number(string=w375) -> (number=w383:dbl)  [unwired: 3 in, 1 out]
        n186 = case shown="\"R\"" w376 {
          tunnel: w383 -> [w386 w404 w421 w427 w434 w440]
          tunnel: w382 -> [w400 w418 w426 w433 w438 w444]
          tunnel: [w399 w417 w426 w433 w438 w444] -> w381
          tunnel: w380 -> [w393 w411 w424 w431 w437 w443]
          tunnel: [w393 w411 w425 w432 w437 w443] -> w379
          tunnel: i16 10000 ("Timeout") -> [w385 w403 w422 w428 _ _]
          tunnel: w372 -> [w384 w402 w420 _ _ w439]
          frame "F" {
            n187 = expression code="(x/180.0)*pi" "degrees to radians"(w393) -> (w396:dbl)
            n188 = Sine(x=w396) -> (sin(x)=w394:dbl)
            n189 = Cosine(x=w396) -> (cos(x)=w395:dbl)
            n190 = Multiply(x=w386, y=w394) -> (x*y=w398:dbl)
            n191 = Multiply(x=w386, y=w395) -> (x*y=w397:dbl)
            n192 = Multiply(x=1250.0, y=w386) -> (x*y=w389:dbl)
            n193 = Bundle(w398, w397) -> (w390:cluster{dbl, dbl})  [unwired: 1 in]
            n194 = call "New PID Move Talon.vi"("Cluster 3"=w384, "Timeout"=w385, "Target Distance"=w389, "Target Angle"=0.0) -> ()  [unwired: 7 in, 1 out]
            n195 = call <vilib>:"Draw Line.vi"("picture"=w400, "end point"=w390, "absolute coordinates?(T)"=FALSE, "color(black)"=u32 6618880, "pen"=T16 {"Width"=2, "Style"=enum."Solid"}) -> ("new picture"=w399:picture)  [unwired: 4 in]
          }
          frame "B" {
            n196 = expression code="(x/180.0)*pi" "degrees to radians"(w411) -> (w414:dbl)
            n197 = Sine(x=w414) -> (sin(x)=w412:dbl)
            n198 = Cosine(x=w414) -> (cos(x)=w413:dbl)
            n199 = Multiply(x=w404, y=w412) -> (x*y=w416:dbl)
            n200 = Multiply(x=w404, y=w413) -> (x*y=w415:dbl)
            n201 = Multiply(x=1250.0, y=w404) -> (x*y=w407:dbl)
            n202 = Bundle(w416, w415) -> (w408:cluster{dbl, dbl})  [unwired: 1 in]
            n203 = call "New PID Move Talon.vi"("Cluster 3"=w402, "Timeout"=w403, "Target Distance"=w407, "Target Angle"=0.0) -> ()  [unwired: 7 in, 1 out]
            n204 = call <vilib>:"Draw Line.vi"("picture"=w418, "end point"=w408, "absolute coordinates?(T)"=FALSE, "color(black)"=u32 6618880, "pen"=T16 {"Width"=2, "Style"=enum."Solid"}) -> ("new picture"=w417:picture)  [unwired: 4 in]
          }
          frame "R" {
            n205 = Subtract(x=w424, y=w421) -> (x-y=w425:dbl)
            n206 = call "New PID Move Talon.vi"("Cluster 3"=w420, "Timeout"=w422, "Target Distance"=0.0, "Target Angle"=w421) -> ()  [unwired: 7 in, 1 out]
          }
          frame "L" {
            n207 = Negate(x=w427) -> (-x=w430:dbl)
            n208 = call "New PID Move Talon.vi"("Timeout"=w428, "Target Distance"=0.0, "Target Angle"=w430) -> ()  [unwired: 8 in, 1 out]
            n209 = Add(x=w431, y=w427) -> (x+y=w432:dbl)
          }
          frame "D", Default {
            n210 = Multiply(x=1000.0, y=w434) -> (x*y=w436:dbl)
            n211 = Wait (ms)(milliseconds to wait=w436) -> ()  [unwired: 1 out]
          }
          frame "C" {
            (unwired) -0.75 ("Power 2")
            (unwired) 0.75 ("Power")
            n212 = Unbundle By Name(w439) -> ("Left Intake"=w442:string, "Right Intake"=w441:string)
            n213 = call "Unguided Move.vi"("milliseconds to wait"=w440, "refnum name 2"=w441, "refnum name"=w442) -> ()  [unwired: 8 in, 1 out]
          }
        }
      }
    }
    frame Enabled {
    }
  }
